vi "2015Swerve_SteeringAdjustment_ActualMath.vi"(9 "Wheel Power":dbl, 10 "Encoder Setpoint":dbl, 11 "Encoder Position":dbl) -> (1 "Wheel Power Out":dbl, 2 "Encoder Setpoint Out":dbl)   [LabVIEW 2014]
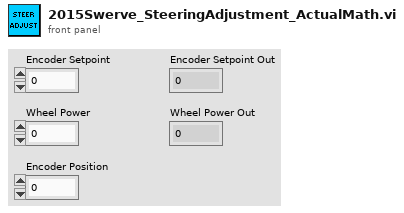
[diagram p1: front panel]
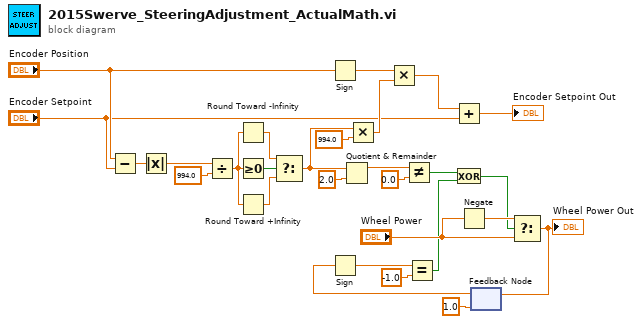
[diagram p0: block diagram]
diagram:
  n1 = Subtract(x="Encoder Position", y="Encoder Setpoint") -> (x-y=w28:dbl)
  n2 = Absolute Value(x=w28) -> (abs(x)=w27:dbl)
  n3 = Divide(x=w27, y=994.0) -> (x/y=w2:dbl)
  n4 = Round Toward -Infinity(1:w2) -> (0:w4:dbl)
  n5 = Greater Or Equal To 0?(x=w2) -> (x >= 0?=w5:bool)
  n6 = Round Toward +Infinity(x=w2) -> (ceil(x): smallest int >= x=w3:dbl)
  n7 = Select(t=w4, s=w5, f=w3) -> (s? t:f=w1:dbl)
  n8 = Sign(1:"Encoder Position") -> (0:w23:dbl)
  n9 = Quotient & Remainder(x=w1, y=2.0) -> (x-y*floor(x/y)=w17:dbl)  [unwired: 1 out]
  n10 = Multiply(x=w1, y=994.0) -> (x*y=w24:dbl)
  n11 = Multiply(x=w23, y=w24) -> (x*y=w21:dbl)
  n12 = Not Equal?(x=w17, y=0.0) -> (x != y?=w8:bool)
  n13 = Add(x=w21, y="Encoder Setpoint") -> (x+y=→"Encoder Setpoint Out":dbl)
  n14 = Negate(x="Wheel Power") -> (-x=w13:dbl)
  n15 = feedback #1(1.0 ("Wheel Power")) -> (w9:dbl)
  n16 = Sign(1:w9) -> (0:w10:dbl)
  n17 = Equal?(x=w10, y=-1.0) -> (x = y?=w7:bool)
  n18 = Exclusive Or(1:w7, 2:w8) -> (0:w6:bool)
  n19 = Select(t=w13, s=w6, f="Wheel Power") -> (s? t:f=w14:dbl)
  "Wheel Power Out" <- w14
  n20 = feedback-in #1(w14) -> ()
